vi "MES操作函数2.vi"(3 "Tips":bool, 5 "测试结果":string="产品名称：SA 左前玻璃升降器\n测试程序版本：150113-A0\n测试时间：\n,,!测试步骤,判定条件,测试值!上电,-,电压：14.0V 限流：1.0A!软件版本号,{06 50 01 00 32 01 F4 AA;\n03 7F 2F 31 AA AA AA AA},06 50 01 00 32 01 F4 AA \n03 7F 2F 31 AA AA AA AA ;!中控锁上锁,{01 AA 02 A4 86 01 01},00 AA 02 A4 86 01 01 90 ，不合格!", 6 "抓图？":bool, 7 "SN":string="0105442MF011400002", 8 "error in (no error)":errorcluster caption="错误输入（无错误）", 9 "二次？":bool, 10 "总结果（测试）":bool, 11 "MES配置":T2={"接口地址："="http://10.9.30.175:50100/manufacturing/IntegrationServlet?InterType=XML&message=", "SITE（站点）   "="A157", "PWD（口令）"="123456", "RESOURCE（资源）"="A-6-Z-TEST", "OPERATION（工序）"="Z-TEST", "USER（用户）"="TEST", "QTY"="", "ACTIVITY"="", "NC_CODE（NG代码）"="", "启用MES"=TRUE}) -> (0 "error out":errorcluster caption="错误输出", 1 "报错?":bool, 2 "Data(OUT)":string="http://10.9.30.175:50100/manufacturing/IntegrationServlet?InterType=XML&message= ERROR<PRODUCTION_REQUEST><NC_LOG_COMPLETE><SITE>A157</SITE><OWNER TYPE=\"USER\">TEST</OWNER><NC_CONTEXT>0105442MF011400002</NC_CONTEXT><QTY></QTY><IDENTIFIER></IDENTIFIER><FAILURE_ID></FAILURE_ID><DEFECT_COUNT>1</DEFECT_COUNT><COMMENTS></COMMENTS><DATE_TIME></DATE_TIME><RESOURCE>A-6-Z-TEST</RESOURCE><OPERATION>Z-TEST</OPERATION><ROOT_CAUSE_OPER></ROOT_CAUSE_OPER><NC_CODE></NC_CODE><ACTIVITY></ACTIVITY></NC_LOG_COMPLETE></PRODUCTION_REQUEST>!erpautogy03!1234567@byd!ERROR,测试文件11V1.0,测试程序11V1.0!产品名称：SA 左前玻璃升降器\n测试程序版本：150113-A0\n测试时间：\n,,!测试步骤,判定条件,测试值!上电,-,电压：14.0V 限流：1.0A!软件版本号,{06 50 01 00 32 01 F4 AA;\n03 7F 2F 31 AA AA AA AA},06 50 01 00 32 01 F4 AA \n03 7F 2F 31 AA AA AA AA ;!中控锁上锁,{01 AA 02 A4 86 01 01},00 AA 02 A4 86 01 01 90 ，不合格!")   [LabVIEW 2011]
panel:
  out "输出簇":T1
  out "数组":string[](array[string])
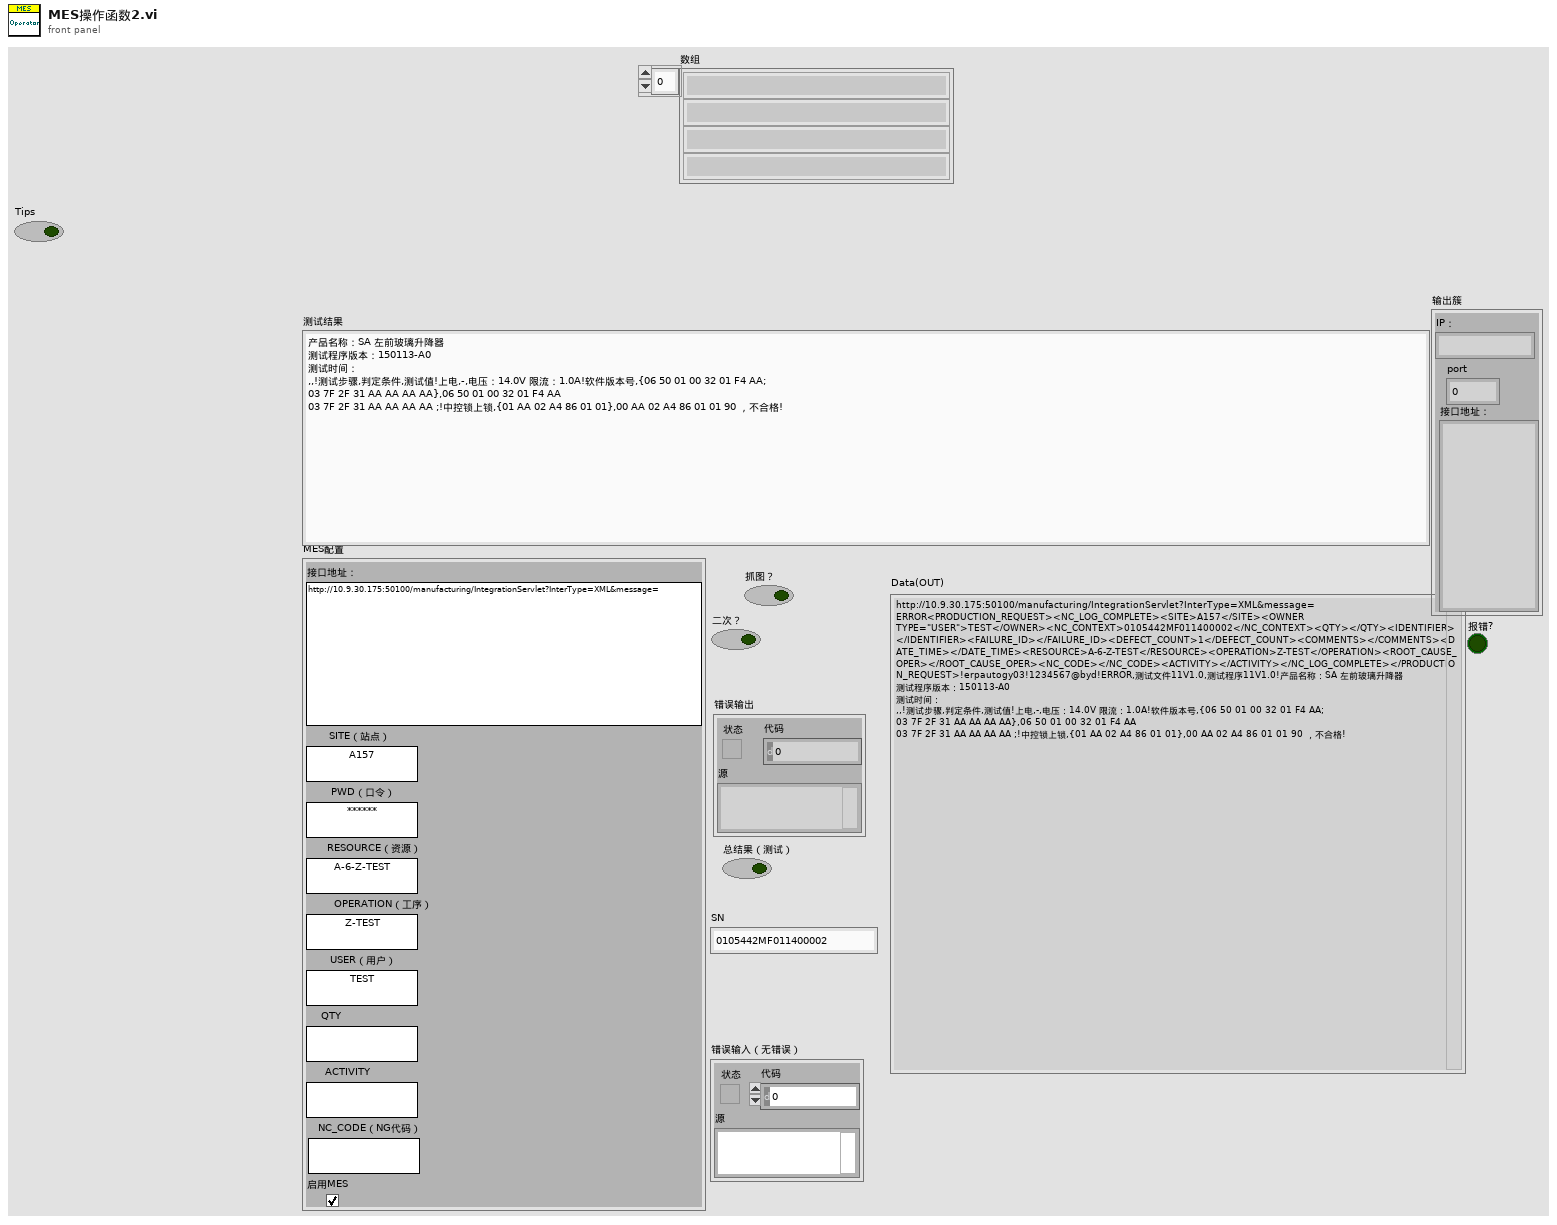
[diagram p1: front panel]
types:
  T1 = cluster{"IP：":string, "port":i32, "接口地址：":string}
  T2 = typedef "MES设置.ctl" = cluster{"接口地址：":string, "SITE（站点）   ":string, "PWD（口令）":string, "RESOURCE（资源）":string, "OPERATION（工序）":string, "USER（用户）":string, "QTY":string, "ACTIVITY":string, "NC_CODE（NG代码）":string, "启用MES":bool}
  T3 = enum16{"USER_CHECK", "SFC_CHECK", "RLT_PASS", "RLT_ERROR", "RES_AREA"}[]
  T4 = enum16{"Left Button", "Center Button", "Right Button", "Window Close"}
  T5 = enum16{"USER_CHECK", "SFC_CHECK", "RLT_PASS", "RLT_ERROR", "RES_AREA"}
  T6 = enum16{"open", "replace", "create", "open or create", "replace or create", "replace or create with confirmation"}
  T7 = typedef "imagedata.ctl" = cluster{"image type":i32, "image depth":i32, "image":u8[], "mask":u8[], "colors":u32[], "Rectangle":cluster{"left":i16, "top":i16, "right":i16, "bottom":i16}}
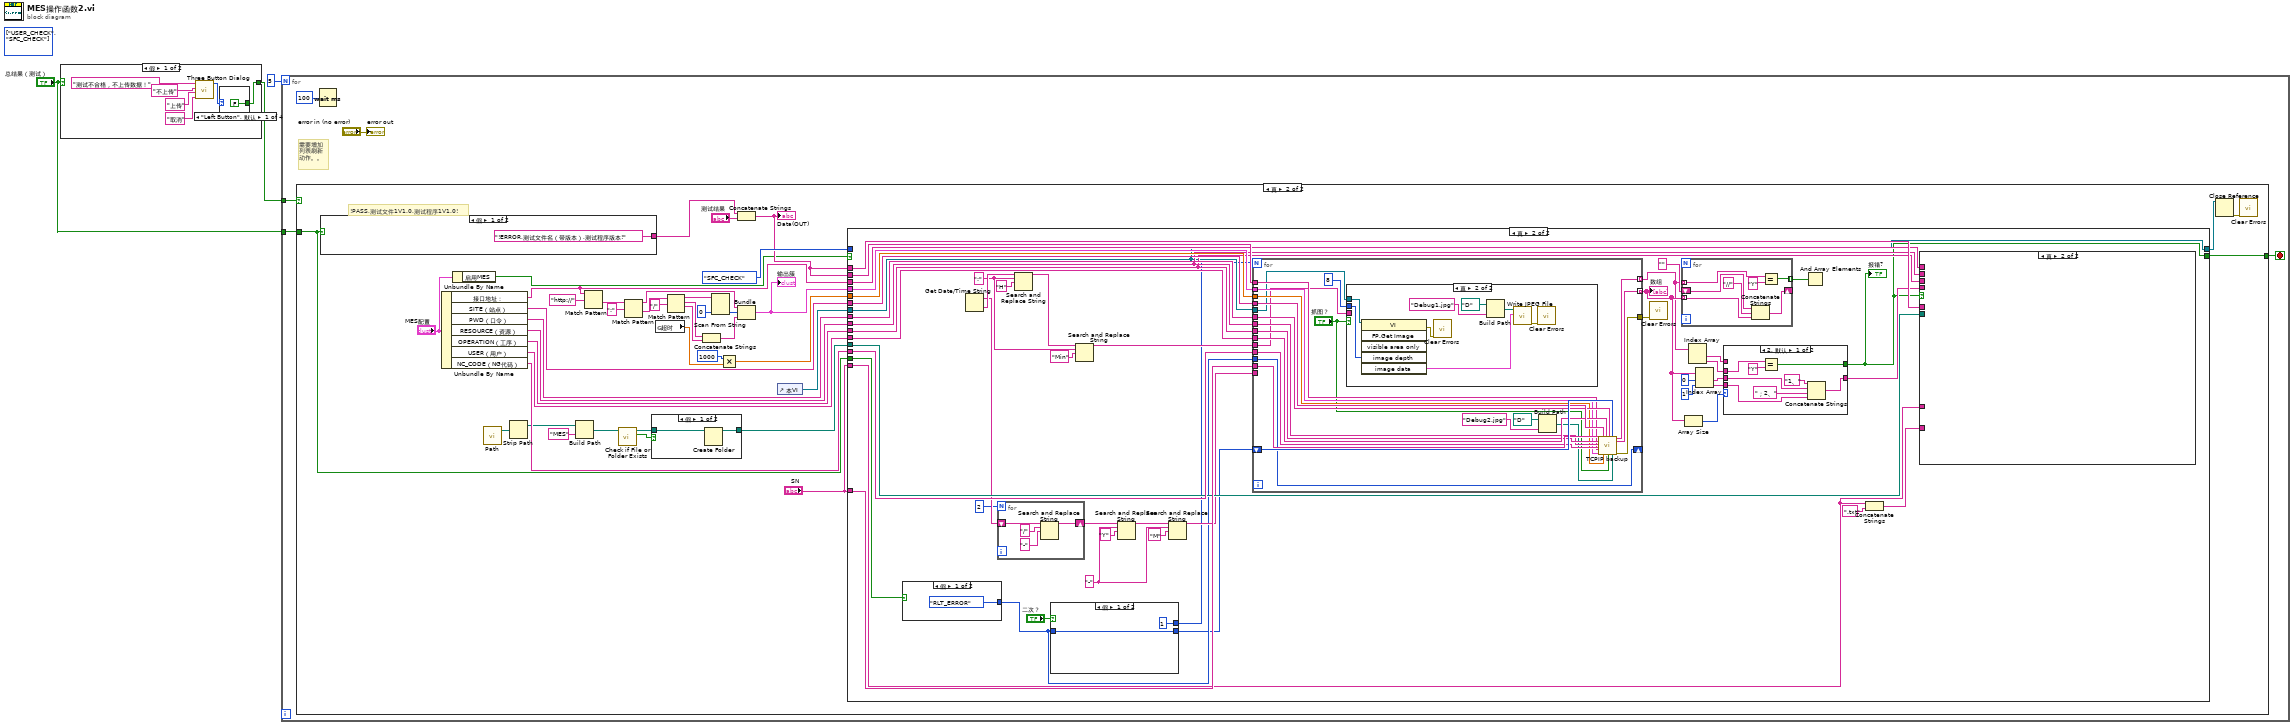
[diagram p0: block diagram]
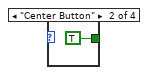
[diagram p2: hidden frame]
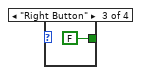
[diagram p3: hidden frame]
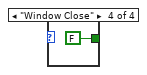
[diagram p4: hidden frame]
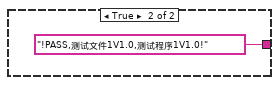
[diagram p8: hidden frame]
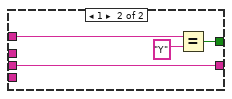
[diagram p10: hidden frame]
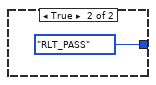
[diagram p11: hidden frame]
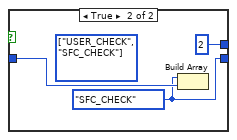
[diagram p12: hidden frame]
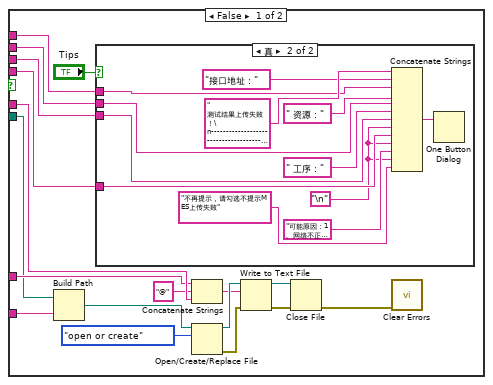
[diagram p13: hidden frame]
diagram:
  (unwired) T3 [enum."USER_CHECK", enum."SFC_CHECK"] items=["USER_CHECK", "SFC_CHECK", "RLT_PASS", "RLT_ERROR", "RES_AREA"]
  n1 = case shown="假" "总结果（测试）" {
    selector: "总结果（测试）" -> [_ w14]
    tunnel: [w4 w14] -> w2
    frame False {
      n2 = call <vilib>:"Three Button Dialog.vi"("Right Button Text (\"Cancel\")"="取消" ("Right Button Text (\"Cancel\")"), "Center Button Text (\"No\")"="上传" ("Center Button Text (\"No\")"), "Left Button Text (\"Yes\")"="不上传" ("Left Button Text (\"Yes\")"), "message"="测试不合格，不上传数据！") -> ("Which Button?"=w5:T4)  [unwired: 7 in]
      n3 = case shown="\"Left Button\", 默认" w5 {
        tunnel: [FALSE TRUE FALSE FALSE] -> w4
        frame "Left Button", Default {
        }
        frame "Center Button" {
        }
        frame "Right Button" {
        }
        frame "Window Close" {
        }
      }
    }
    frame True {
    }
  }
  n4 = for {
    N: 5 -> [_]
    tunnel: w2 -> [w16]
    tunnel: "总结果（测试）" -> [w15]
    stop <- w18 stop-if-true
    # "需要增加\n列表刷新\n动作。。"
    n5 = case shown="真" w16 {
      tunnel: w15 -> [_ w42]
      tunnel: [_ w20] -> w18
      frame False {
      }
      frame True {
        # "!PASS,测试文件1V1.0,测试程序1V1.0!"
        n6 = case shown="假" w42 {
          tunnel: ["!ERROR,测试文件名（带版本）,测试程序版本!" ("字符串") "!PASS,测试文件1V1.0,测试程序1V1.0!" ("字符串")] -> w41
          frame False {
          }
          frame True {
          }
        }
        n7 = Unbundle By Name("MES配置") -> ("接口地址："=w38:string, "SITE（站点）"=w59:string, "PWD（口令）"=w57:string, "RESOURCE（资源）"=w37:string, "OPERATION（工序）"=w56:string, "USER（用户）"=w58:string, "NC_CODE（NG代码）"=w55:string)
        n8 = Unbundle By Name("MES配置") -> ("启用MES"=w26:bool)
        n9 = call "Path.vi"() -> ("appended path"=w31:path)  [unwired: 11 in]
        n10 = Strip Path(path=w31) -> (stripped path=w32:path)  [unwired: 1 out]
        n11 = Build Path(base path=w32, name or relative path="MES" ("名称或相对路径")) -> (appended path=w34:path)
        n12 = Match Pattern(string=w38, regular expression="http://" ("正则表达式")) -> (after substring=w51:string)  [unwired: 1 in, 3 out]
        n13 = call <vilib>:"Check if File or Folder Exists.vi"("path"=w34) -> ("file or folder exists?"=w35:bool, "dup path"=w36:path)  [unwired: 8 in, 1 out]
        n14 = Match Pattern(string=w51, regular expression=":" ("正则表达式")) -> (before substring=w46:string, after substring=w49:string)  [unwired: 1 in, 2 out]
        n15 = case shown="假" w35 {
          tunnel: w36 -> [w62 w64]
          tunnel: [w63 w64] -> w30
          frame False {
            n16 = Create Folder(path (use dialog)=w62) -> (created path=w63:path)  [unwired: 2 in, 2 out]
          }
          frame True {
          }
        }
        n17 = global read "全局 TCPIP超时.vi" "超时"() -> (w21:dbl)
        n18 = Match Pattern(string=w49, regular expression="/" ("正则表达式")) -> (before substring=w47:string, match substring=w23:string, after substring=w25:string)  [unwired: 1 in, 1 out]
        n19 = Concatenate Strings(w23, w25) -> (w24:string)
        n20 = Scan From String(input string=w47, default 1=0 ("默认值 1")) -> (output 1=w44:i32)  [unwired: 3 in, 3 out]
        n21 = Multiply(x=u64 1000 ("TCP超时"), y=w21) -> (x*y=w22:dbl)
        n22 = Concatenate Strings(w41, "测试结果") -> (w40:string)
        "Data(OUT)" <- w40
        n23 = Bundle("接口地址："=w46, "默认值 1"=w44, w24) -> (w45:cluster{"接口地址：":string, "默认值 1":i32, string})  [unwired: 1 in]
        "输出簇" <- w45
        n24 = control-ref of="本VI"() -> (w29:refnum<vi>)
        n25 = case shown="真" w26 {
          tunnel: T5."SFC_CHECK" ("STATE") -> [_ _]
          tunnel: w59 -> [_ w117]
          tunnel: w58 -> [_ w116]
          tunnel: w57 -> [_ w115]
          tunnel: "SN" -> [_ w114]
          tunnel: w56 -> [_ w93]
          tunnel: w55 -> [_ w113]
          tunnel: w22 -> [_ w112]
          tunnel: w40 -> [_ w111]
          tunnel: w45 -> [_ w110]
          tunnel: w42 -> [_ w82]
          tunnel: w40 -> [_ w107]
          tunnel: "SN" -> [_ w85]
          tunnel: w38 -> [_ w95]
          tunnel: w37 -> [_ w94]
          tunnel: w29 -> [w67 w89]
          tunnel: w30 -> [_ w92]
          tunnel: [w67 w89] -> w28
          tunnel: [_ w68] -> w20
          frame False {
          }
          frame True {
            w103 = ":" ("搜索字符串")
            w100 = "-" ("搜索字符串")
            n26 = case shown="假" w82 {
              tunnel: [T5."RLT_ERROR" ("STATE") T5."RLT_PASS" ("STATE")] -> w81
              frame False {
              }
              frame True {
              }
            }
            n27 = Get Date/Time String() -> (date string=w88:string, time string=w106:string)  [unwired: 3 in]
            n28 = for {
              N: 2 -> [_]
              shift-right: [w137] -> w86
              shift-left: w88 -> [w140]
              n29 = Search and Replace String(input string=w140, search string="/" ("搜索字符串"), replace string="-" ("替换字符串(\"\")")) -> (result string=w137:string)  [unwired: 5 in, 3 out]
            }
            n30 = Search and Replace String(input string=w106, search string=w103, replace string="H" ("替换字符串(\"\")")) -> (result string=w104:string)  [unwired: 5 in, 3 out]
            n31 = case shown="假" "二次？" {
              tunnel: [1 2] -> w70
              tunnel: w81 -> [w132 w135]
              tunnel: [w132 w134] -> w69
              frame False {
              }
              frame True {
                (unwired) T3 [enum."USER_CHECK", enum."SFC_CHECK"] items=["USER_CHECK", "SFC_CHECK", "RLT_PASS", "RLT_ERROR", "RES_AREA"]
                w134 = T5."SFC_CHECK" ("STATE")
                n32 = Build Array(w134, w135) -> ()  [unwired: 1 out]
              }
            }
            n33 = Search and Replace String(input string=w104, search string=w103, replace string="Min" ("替换字符串(\"\")")) -> (result string=w90:string)  [unwired: 5 in, 3 out]
            n34 = Search and Replace String(input string=w86, search string=w100, replace string="Y" ("替换字符串(\"\")")) -> (result string=w99:string)  [unwired: 5 in, 3 out]
            n35 = Search and Replace String(input string=w99, search string=w100, replace string="M" ("替换字符串(\"\")")) -> (result string=w91:string)  [unwired: 5 in, 3 out]
            n36 = for {
              N: w70 -> [_]
              tunnel: w117 -> [w198]
              tunnel: w116 -> [w197]
              tunnel: w115 -> [w196]
              tunnel: w114 -> [w195]
              tunnel: w93 -> [w194]
              tunnel: w94 -> [w193]
              tunnel: w113 -> [w192]
              tunnel: w112 -> [w191]
              tunnel: w111 -> [w190]
              tunnel: w110 -> [w189]
              tunnel: [w188] -> w80 mode=indexing
              tunnel: [w187] -> w76 mode=indexing
              tunnel: [w186] -> w96
              tunnel: w89 -> [w185]
              tunnel: w91 -> [_]
              tunnel: w90 -> [w183]
              tunnel: w81 -> [w178]
              shift-right: [w178] -> _
              shift-left: w69 -> [w199]
              n37 = case shown="真" "抓图？" {
                tunnel: w185 -> [_ w207]
                tunnel: 8 ("图像深度") -> [_ w206]
                tunnel: w183 -> [_ _]
                frame False {
                }
                frame True {
                  n38 = invoke class="VI" method="FP.Get Image"(reference=w207, "image depth"=w206) -> (error out=w204:errorcluster, "image data"=w205:T7)  [unwired: 4 in, 4 out]
                  n39 = call <vilib>:"Clear Errors.vi"("error in (no error)"=w204) -> ()  [unwired: 6 in, 1 out]
                  n40 = Build Path(base path=path "D:/" ("基路径"), name or relative path="Debug1.jpg" ("名称或相对路径")) -> (appended path=w203:path)
                  n41 = call <vilib>:"Write JPEG File.vi"("image data"=w205, "path to JPEG file"=w203) -> ("error out"=w202:errorcluster)  [unwired: 8 in, 1 out]
                  n42 = call <vilib>:"Clear Errors.vi"("error in (no error)"=w202) -> ()  [unwired: 6 in, 1 out]
                }
              }
              n43 = Build Path(base path=path "D:/" ("基路径"), name or relative path="Debug2.jpg" ("名称或相对路径")) -> (appended path=w179:path)
              n44 = call "TCPIP backup.vi"("SFC"=w195, "OPERATOR"=w194, "RESOURCE"=w193, "NC_CODE"=w192, "TESTRLT"=w190, "SERVER"=w189, "SITE"=w198, "TCP超时"=w191, "USER"=w197, "PWD"=w196, "抓图？"="抓图？", "STATE"=w199, "path to JPEG file"=w179) -> ("Y&N"=w187:string, "系统消息"=w188:string, "error out"=w186:errorcluster)  [unwired: 4 in]
            }
            "数组" <- w80
            n45 = call <vilib>:"Clear Errors.vi"("error in (no error)"=w96) -> ()  [unwired: 6 in, 1 out]
            n46 = for {
              tunnel: w76 -> [w177] mode=indexing
              tunnel: [w175] -> w109 mode=indexing
              tunnel: w80 -> [w174] mode=indexing
              shift-right: [w173] -> _
              shift-left: "" -> [w172]
              n47 = Concatenate Strings(w172, "//" ("字符串"), w174) -> (w173:string)
              n48 = Equal?(x=w177, y="Y") -> (x = y?=w175:bool)
            }
            n49 = Array Size(array=w80) -> (size(s)=w77:i32)
            n50 = Index Array(array=w76) -> (element #1=w75:string, element #2=w74:string)  [unwired: 2 in]
            n51 = Index Array(array=w80, index #1=0 ("索引"), index #2=1 ("索引")) -> (element #1=w73:string, element #2=w71:string)
            n52 = case shown="2, 默认" w77 {
              tunnel: w75 -> [_ w128]
              tunnel: w74 -> [w123 _]
              tunnel: [w124 w127] -> w68
              tunnel: [w118 w126] -> w72
              tunnel: w73 -> [w121 w126]
              tunnel: w71 -> [w122 _]
              frame 2, Default {
                n53 = Equal?(x=w123, y="Y") -> (x = y?=w124:bool)
                n54 = Concatenate Strings("1、" ("字符串"), w121, "；2、" ("字符串"), w122) -> (w118:string)
              }
              frame 1 {
                n55 = Equal?(x=w128, y="Y") -> (x = y?=w127:bool)
              }
            }
            "报错?" <- w68
            n56 = And Array Elements(Boolean array=w109) -> ()  [unwired: 1 out]
            n57 = Concatenate Strings(w85, ".txt" ("字符串")) -> (w84:string)
            n58 = case shown="真" w68 {
              tunnel: w72 -> [w158 _]
              tunnel: w107 -> [w149 _]
              tunnel: w85 -> [w148 _]
              tunnel: w95 -> [w145 _]
              tunnel: w94 -> [w144 _]
              tunnel: w93 -> [w143 _]
              tunnel: w92 -> [w142 _]
              tunnel: w84 -> [w141 _]
              frame False {
                n59 = Build Path(base path=w142, name or relative path=w141) -> (appended path=w156:path)
                n60 = case shown="真" "Tips" {
                  tunnel: w158 -> [_ w169]
                  tunnel: w145 -> [_ w163]
                  tunnel: w144 -> [_ w161]
                  tunnel: w143 -> [_ w159]
                  frame False {
                  }
                  frame True {
                    w167 = "\n"
                    n61 = Concatenate Strings("                  测试结果上传失败！\n---------------------------------------------\n", "接口地址：" ("字符串"), w163, " 资源：" ("字符串"), w161, " 工序：" ("字符串"), w159, w167, w169, w167, "可能原因：1、网络不正确；2、配置参数错误；3、条码错误；4、SFC未维护。" ("字符串"), w167, "不再提示，请勾选不提示MES上传失败" ("字符串")) -> (w170:string)
                    n62 = One Button Dialog(message=w170) -> ()  [unwired: 1 in, 1 out]
                  }
                }
                n63 = Concatenate Strings(w148, "@" ("字符串"), w149) -> (w146:string)
                n64 = Open/Create/Replace File(file path (use dialog)=w156, operation (0:open)=T6."open or create" ("操作(0:open)")) -> (refnum out=w154:refnum<file>, error out=w153:errorcluster)  [unwired: 4 in, 1 out]
                n65 = Write to Text File(file (use dialog)=w154, text=w146, error in=w153) -> (refnum out=w151:refnum<file>, error out=w152:errorcluster)  [unwired: 1 in, 1 out]
                n66 = Close File(refnum=w151, error in=w152) -> (error out=w150:errorcluster)  [unwired: 1 out]
                n67 = call <vilib>:"Clear Errors.vi"("error in (no error)"=w150) -> ()  [unwired: 6 in, 1 out]
              }
              frame True {
              }
            }
          }
        }
        n68 = Close Reference(reference=w28) -> (error out=w27:errorcluster)  [unwired: 1 in]
        n69 = call <vilib>:"Clear Errors.vi"("error in (no error)"=w27) -> ()  [unwired: 6 in, 1 out]
      }
    }
    n70 = Wait (ms)(milliseconds to wait=u32 100 ("等待时间（毫秒）")) -> ()  [unwired: 1 out]
    "error out" <- "error in (no error)"
  }
